vi "Edit LakeShore 336.vi"(8 "error in (no error)":errorcluster, 11 "Instrument parameters in":T1) -> (0 "error out":errorcluster, 3 "Instrument parameters out":T1)   [LabVIEW 2025]
panel:
  in  "Wait Time (s)":i32
  in  "Ramp Rate (K/min)":dbl
  in  "Precison (K)":dbl
  in  "Time out (s)":i32
  in  "Ramp":bool
  in  "Update?":bool
  # "LakeShore 336: Settings"
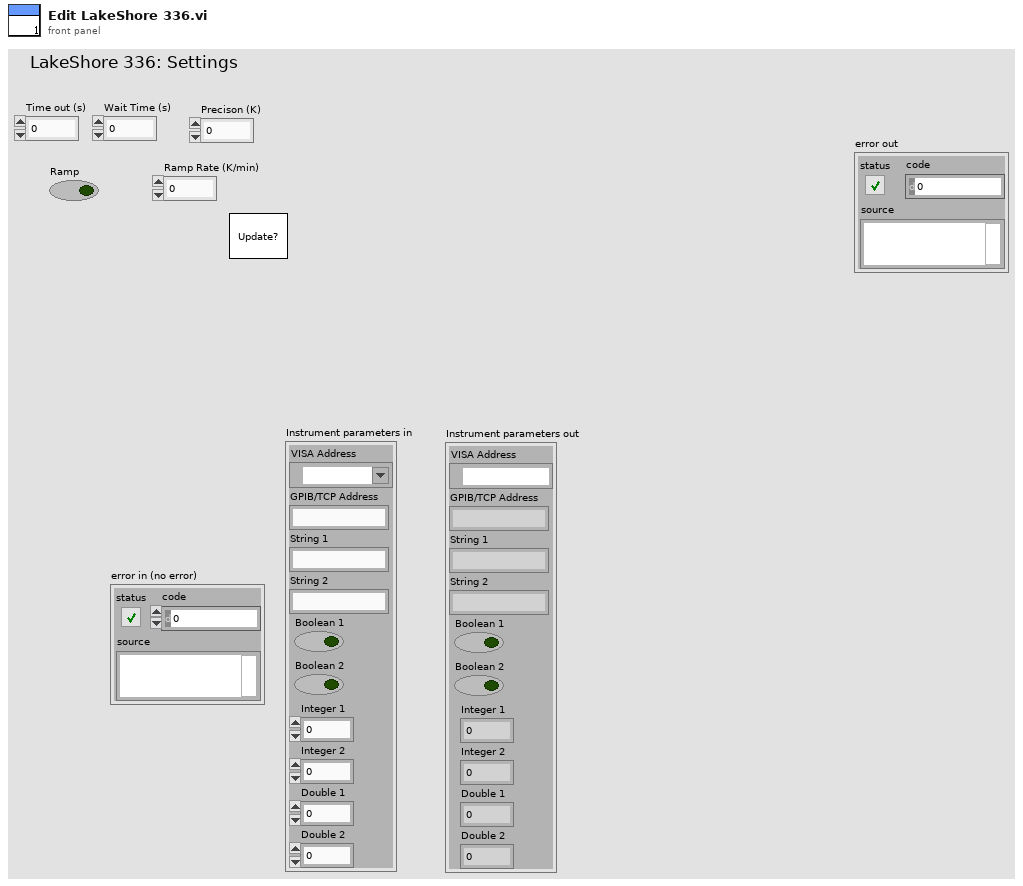
[diagram p1: front panel]
types:
  T1 = cluster{"VISA Address":refnum<visa-resource-name>, "GPIB/TCP Address":string, "String 1":string, "String 2":string, "Boolean 1":bool, "Boolean 2":bool, "Integer 1":i32, "Integer 2":i32, "Double 1":dbl, "Double 2":dbl}
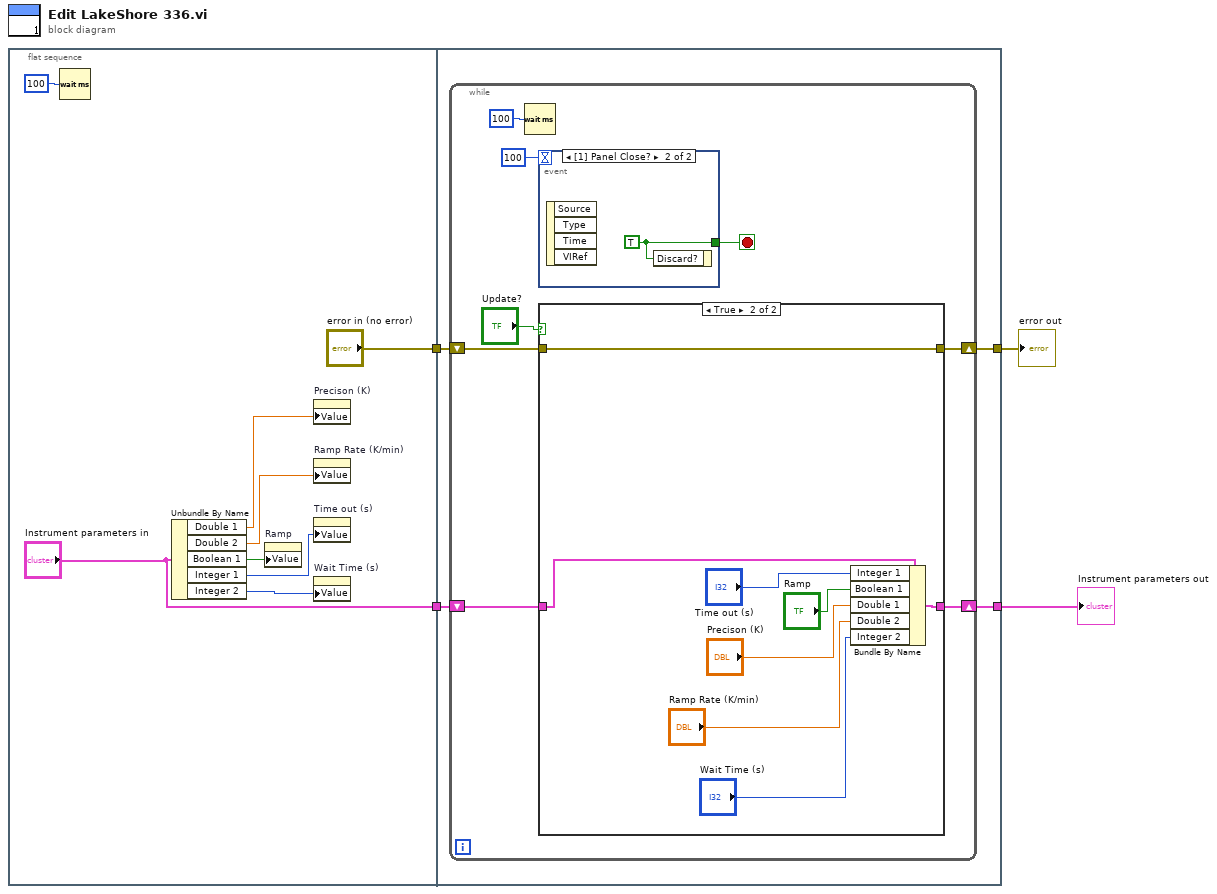
[diagram p0: block diagram]
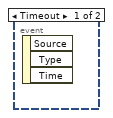
[diagram p3: hidden frame]
diagram:
  n1 = flat-sequence {
    tunnel: ["Instrument parameters in"] -> w4
    tunnel: ["error in (no error)"] -> w2
    tunnel: w4 -> [w16]
    tunnel: [w15] -> w3
    tunnel: w2 -> [w14]
    tunnel: [w13] -> w1
    frame #0 {
      n2 = Wait (ms)(milliseconds to wait=u32 100) -> ()  [unwired: 1 out]
      n3 = Unbundle By Name("Instrument parameters in") -> ("Double 1"=w9:dbl, "Double 2"=w8:dbl, "Boolean 1"=w7:bool, "Integer 1"=w6:i32, "Integer 2"=w5:i32)
      n4 = property on="Ramp" class="Bool (strict)"("Value"=w7) -> ()  [unwired: 2 in, 2 out]
      n5 = property on="Precison (K)" class="DigNum (strict)"("Value"=w9) -> ()  [unwired: 2 in, 2 out]
      n6 = property on="Ramp Rate (K/min)" class="DigNum (strict)"("Value"=w8) -> ()  [unwired: 2 in, 2 out]
      n7 = property on="Time out (s)" class="DigNum (strict)"("Value"=w6) -> ()  [unwired: 2 in, 2 out]
      n8 = property on="Wait Time (s)" class="DigNum (strict)"("Value"=w5) -> ()  [unwired: 2 in, 2 out]
    }
    frame #1 {
      n9 = while {
        shift-right: [w23] -> w15
        shift-left: w16 -> [w18]
        shift-right: [w20] -> w13
        shift-left: w14 -> [w17]
        stop <- w22 stop-if-true
        n10 = Wait (ms)(milliseconds to wait=u32 100) -> ()  [unwired: 1 out]
        n11 = event shown="[1] Panel Close?" {
          selector: _ -> [_ _]
          dyn-events: _ -> [_ _]
          timeout: 100 -> [_ _]
          tunnel: [_ w35] -> w22
          event Timeout {
            n12 = event-data() -> ()  [unwired: 1 in, 3 out]
          }
          event Panel Close? {
            w35 = TRUE ("Discard?")
            n13 = event-data() -> ()  [unwired: 1 in, 4 out]
            n14 = event-data("Discard?"=w35) -> ()  [unwired: 1 in, 1 out]
          }
        }
        n15 = case shown="True" "Update?" {
          tunnel: [w26 w33] -> w23
          tunnel: [w25 w32] -> w20
          tunnel: w18 -> [w26 w34]
          tunnel: w17 -> [w25 w32]
          frame False {
          }
          frame True {
            n16 = Bundle By Name(cluster=w34, "Integer 1"="Time out (s)", "Boolean 1"="Ramp", "Double 1"="Precison (K)", "Double 2"="Ramp Rate (K/min)", "Integer 2"="Wait Time (s)") -> (w33:T1)
          }
        }
      }
    }
  }
  "Instrument parameters out" <- w3
  "error out" <- w1
